vi "Shutdown.vi"(8 "error in (no error)":errorcluster, 11 "Application in":refnum<class "Application.lvclass">) -> (0 "error out":errorcluster, 3 "Application out":refnum<class "Application.lvclass">)   [LabVIEW 2019, in "Application.lvclass"]
doc: "Developed by Kevin Thompson\nkevin@thompsonengineering.net\n\nCopyright 2018\nThompson Engineering, LLC"
uses:
  Application.lvclass
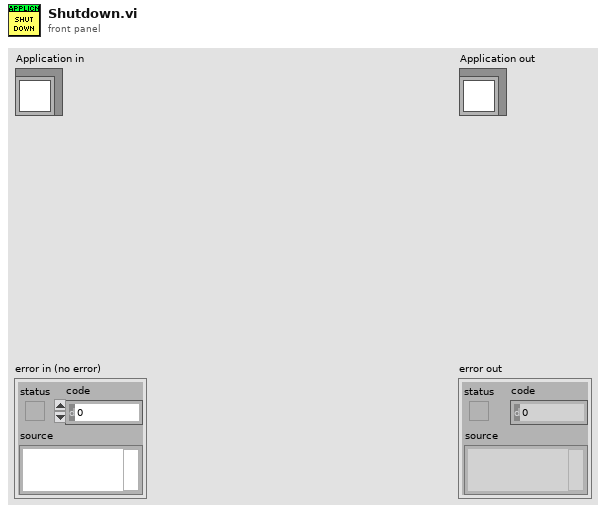
[diagram p1: front panel]
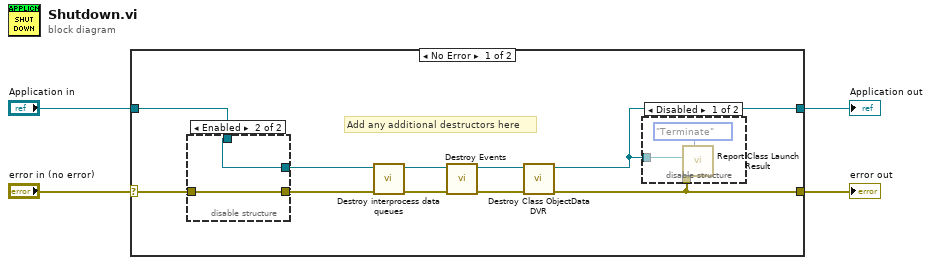
[diagram p0: block diagram]
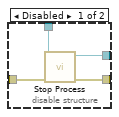
[diagram p3: hidden frame]
diagram:
  n1 = case shown="No Error" "error in (no error)" {
    selector: "error in (no error)" -> [w14 w25]
    tunnel: [w8 w25] -> w3
    tunnel: [w9 w24] -> w1
    tunnel: "Application in" -> [w12 w24]
    frame No Error {
      # "Add any additional destructors here"
      n2 = disable-structure shown="Enabled" {
        disable-tunnel: w14 -> [w21 w22]
        disable-tunnel: [w20 w22] -> w13
        disable-tunnel: w12 -> [w19 w23]
        disable-tunnel: [w18 w23] -> w5
        frame Disabled {
          n3 = call "Stop Process.vi"("error in (no error)"=w21, "Application in"=w19) -> ("error out"=w20:errorcluster, "Application out"=w18:refnum<class "Application.lvclass">)  [unwired: 8 in]
        }
        frame Enabled {
        }
      }
      n4 = call "Destroy interprocess data queues.vi"("error in (no error)"=w13, "Application in"=w5) -> ("error out"=w7:errorcluster, "Application out"=w6:refnum<class "Application.lvclass">)  [unwired: 8 in]
      n5 = call "Destroy Events.vi"("error in (no error)"=w7, "Application in"=w6) -> ("error out"=w11:errorcluster, "Application out"=w10:refnum<class "Application.lvclass">)  [unwired: 8 in]
      n6 = call "Destroy Class ObjectData DVR.vi"("error in (no error)"=w11, "Application in"=w10) -> ("error out"=w8:errorcluster, "Application out"=w9:refnum<class "Application.lvclass">)  [unwired: 8 in]
      n7 = disable-structure shown="Disabled" {
        disable-tunnel: w9 -> [w16 _]
        disable-tunnel: w8 -> [w15 _]
        frame Disabled {
          n8 = call "Report Class Launch Result.vi"("Object"=w16, "error in (no error)"=w15, "Mode (Launch)"=enum16{"Launch", "Terminate"}."Terminate") -> ()  [unwired: 7 in, 1 out]
        }
        frame Enabled {
        }
      }
    }
    frame Error {
    }
  }
  "error out" <- w3
  "Application out" <- w1
